vi "Inst Calibration.vi"() -> ()   [LabVIEW 2016, in "User Interface.lvlib"]
uses:
  User Interface.lvlib
  VI Name.ctl
  Calibration/Calibration.lvlib
  Calibration/Calibration Command.ctl
  Inst Calibration Data Highway.ctl
panel:
  in  "Calibration Check?":bool
  out "Status":string
  in  "Data":string[][](table)
  in  "Save":bool
  in  "Restore":bool
  out "Status":string
  in  "Exit":bool
  in  "Stop":bool
  out "error out":errorcluster
  in  "error in (no error)":errorcluster
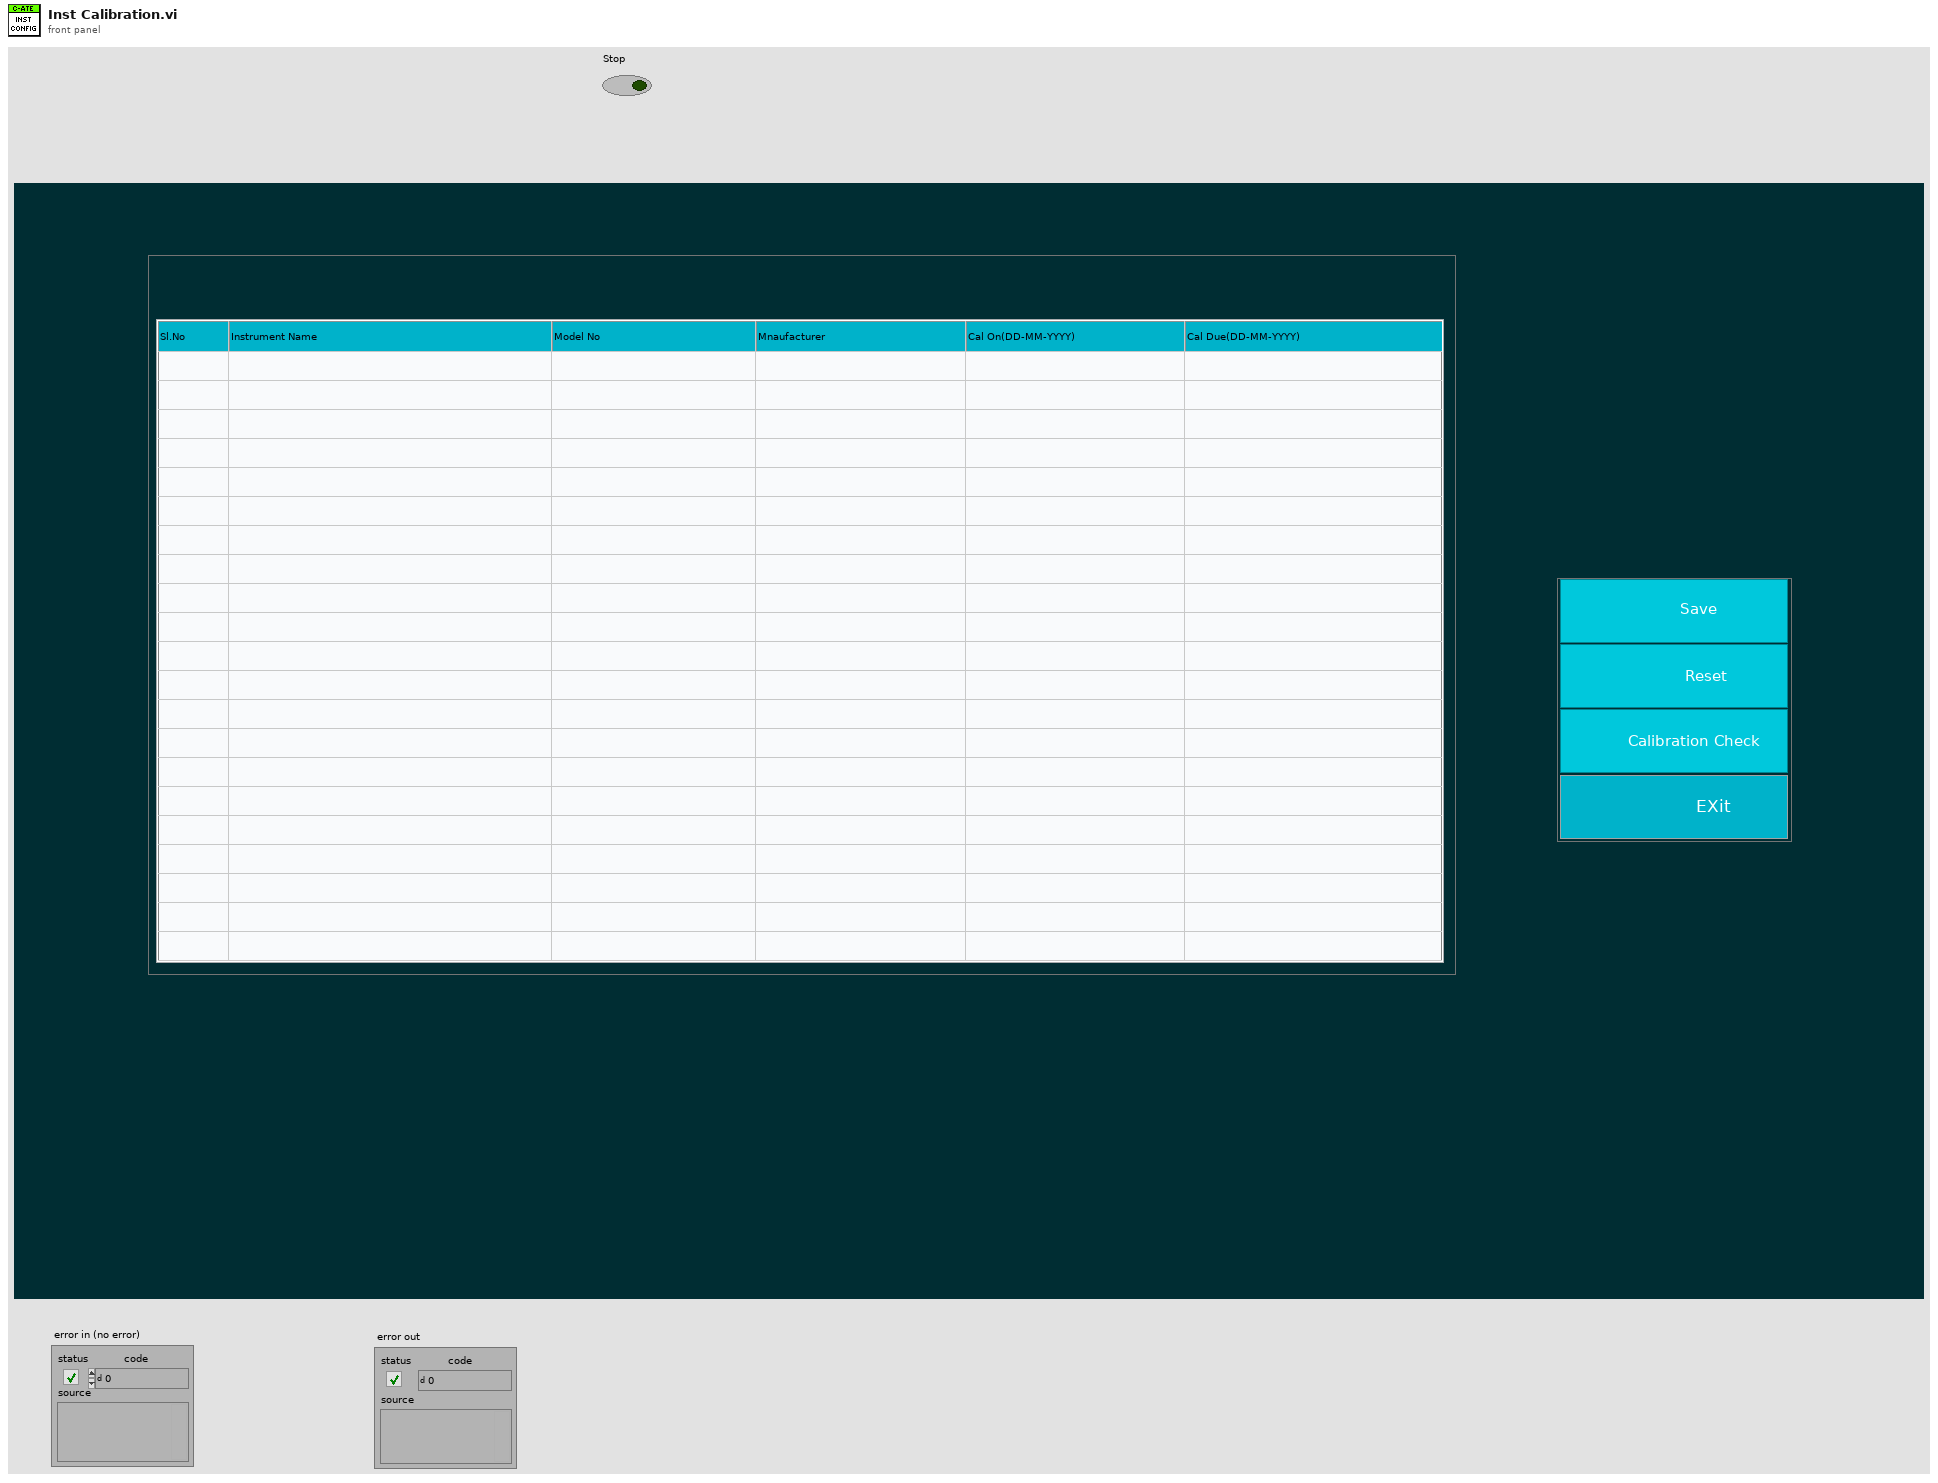
[diagram p1: front panel]
types:
  T1 = typedef "User Interface.lvlib/Inst Calibration Data Highway.ctl" = cluster{"Data":refnum<vi>, "Status":refnum<vi>, "Status":string, "Calibration Due Status":string[]}
  T2 = typedef "Calibration.lvlib/Calibration Command.ctl" = enum16{"Init", "Read", "Write", "Check Calibration", "Close"}
  T3 = typedef "User Interface.lvlib/VI Name.ctl" = enum16{"Dashboard", "Maintenance", "Recipe", "Inst Calibration", "Testing", "Report"}
  T4 = typedef "LVPoint32TypeDef.ctl" = cluster{"Horizontal":i32, "Vertical":i32}
  T5 = typedef "LVRowAndColumnTypeDef.ctl" = cluster{"Row":i32, "Column":i32}
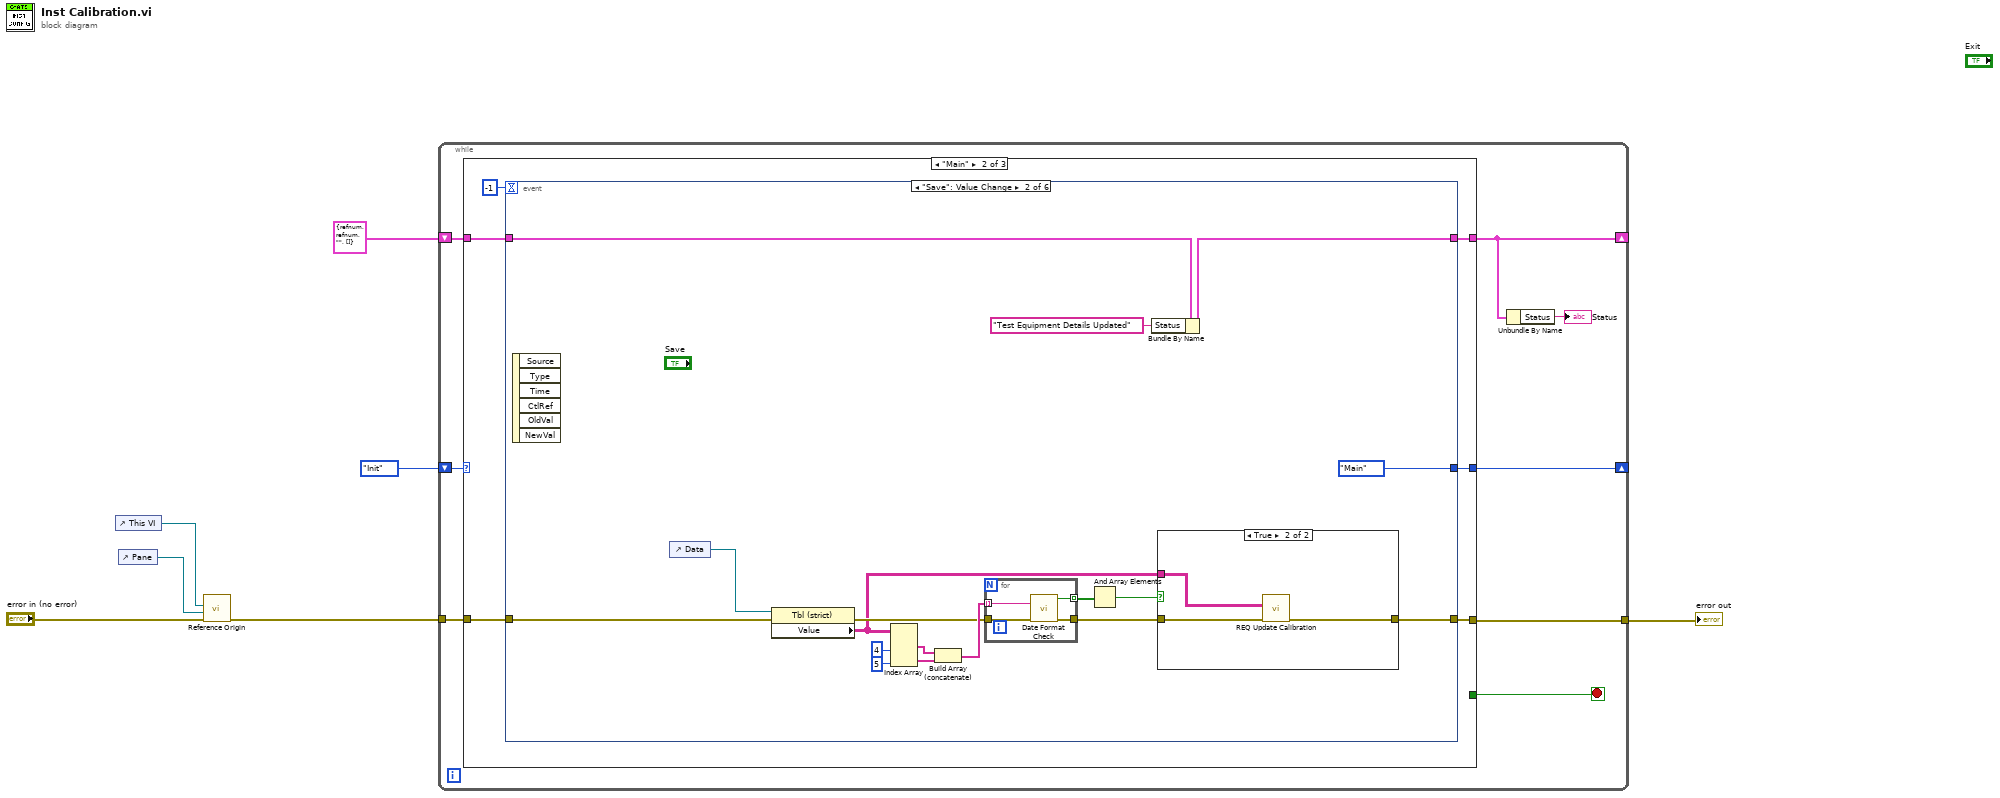
[diagram p0: block diagram]
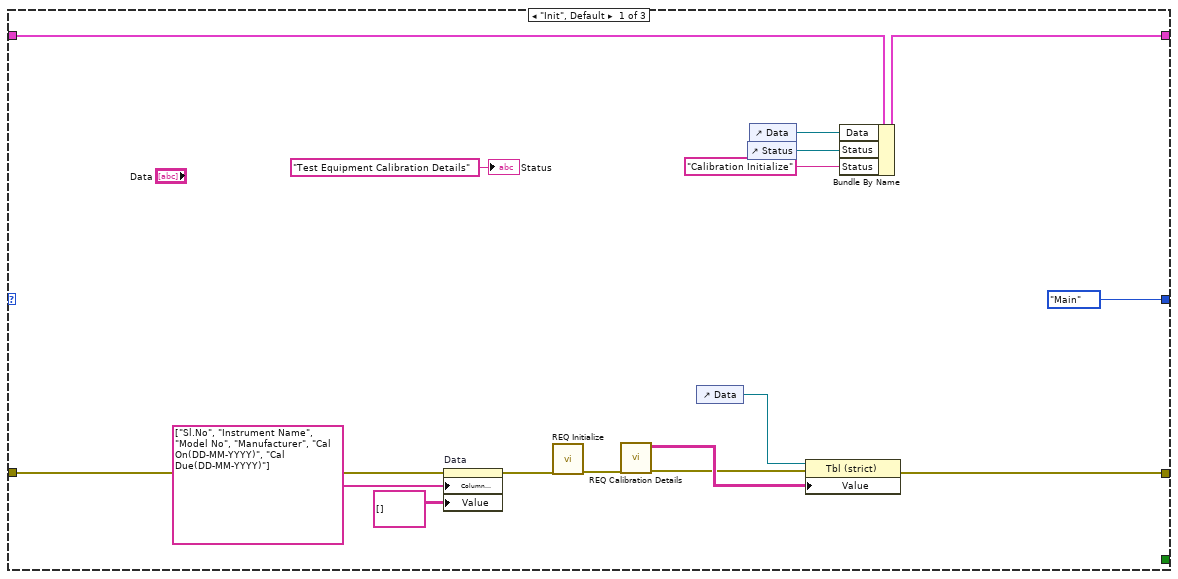
[diagram p2: hidden frame]
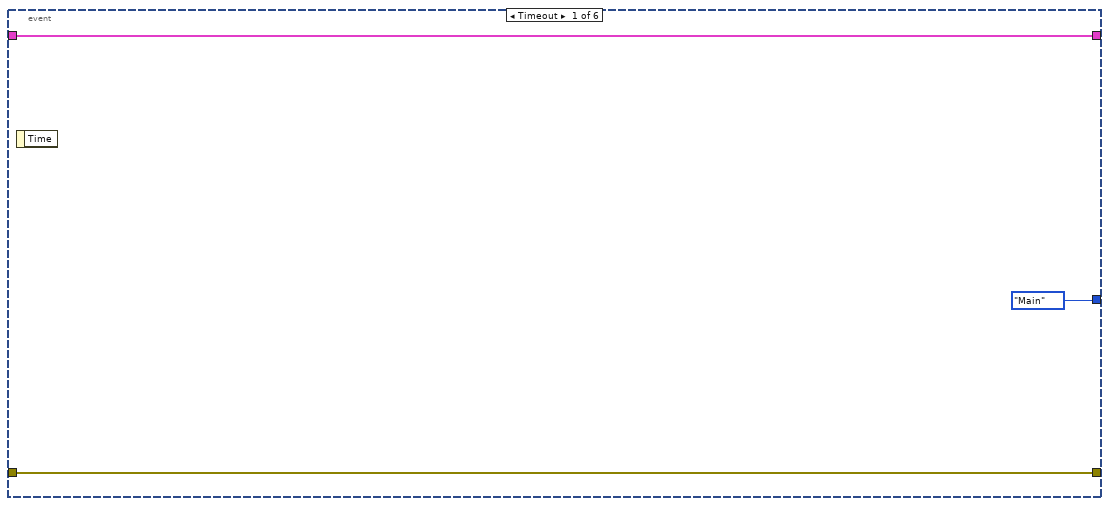
[diagram p3: hidden frame]
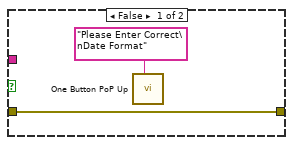
[diagram p4: hidden frame]
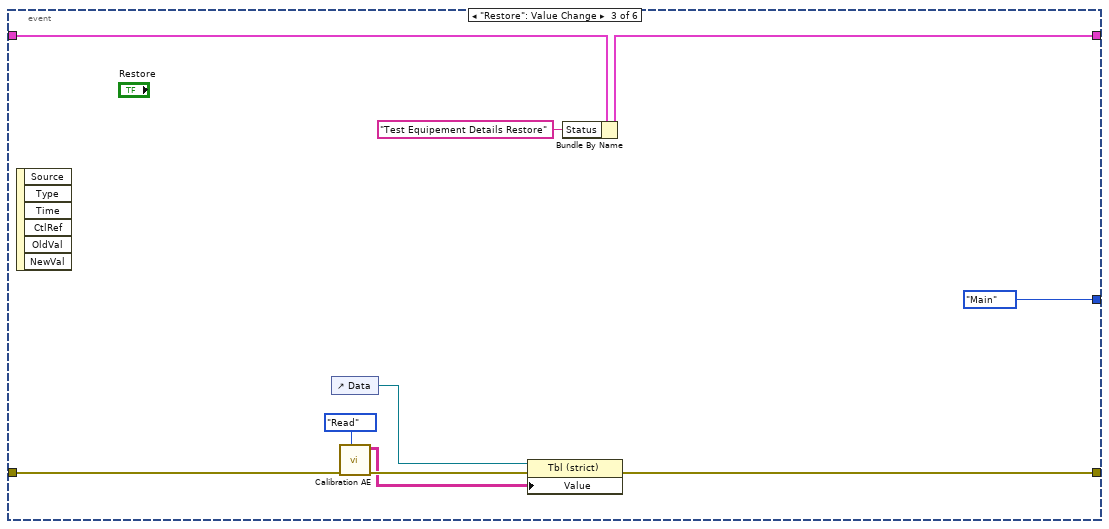
[diagram p5: hidden frame]
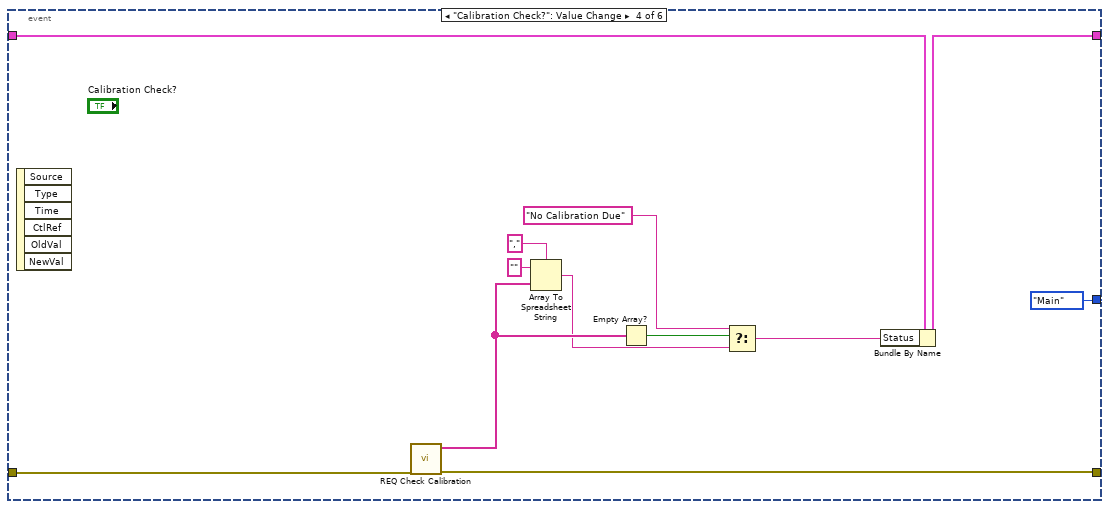
[diagram p6: hidden frame]
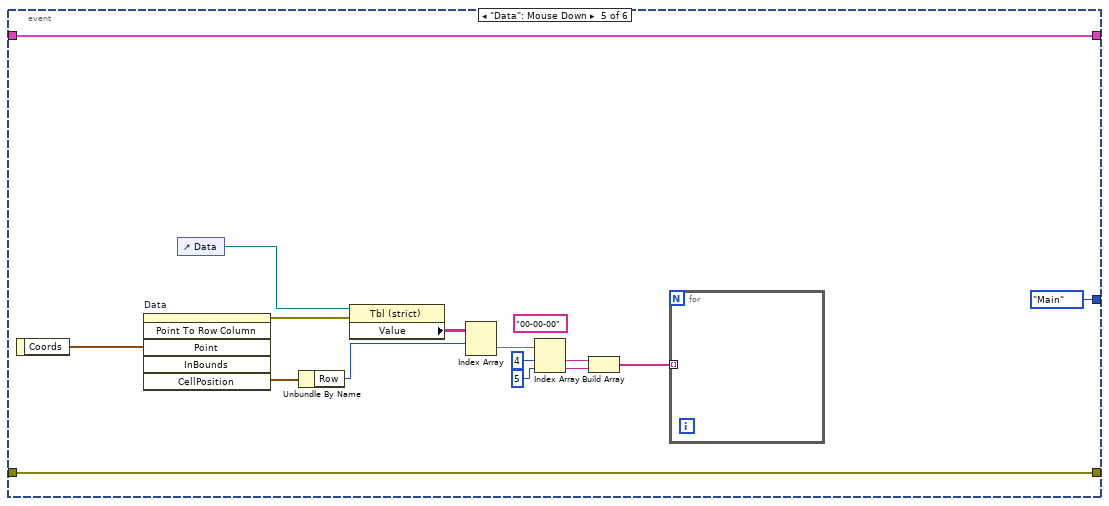
[diagram p7: hidden frame]
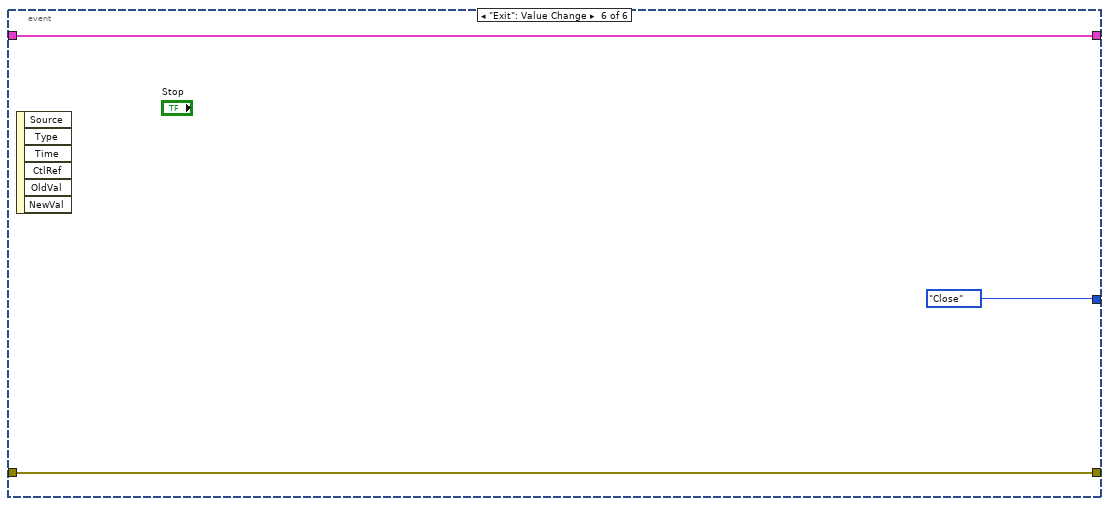
[diagram p8: hidden frame]
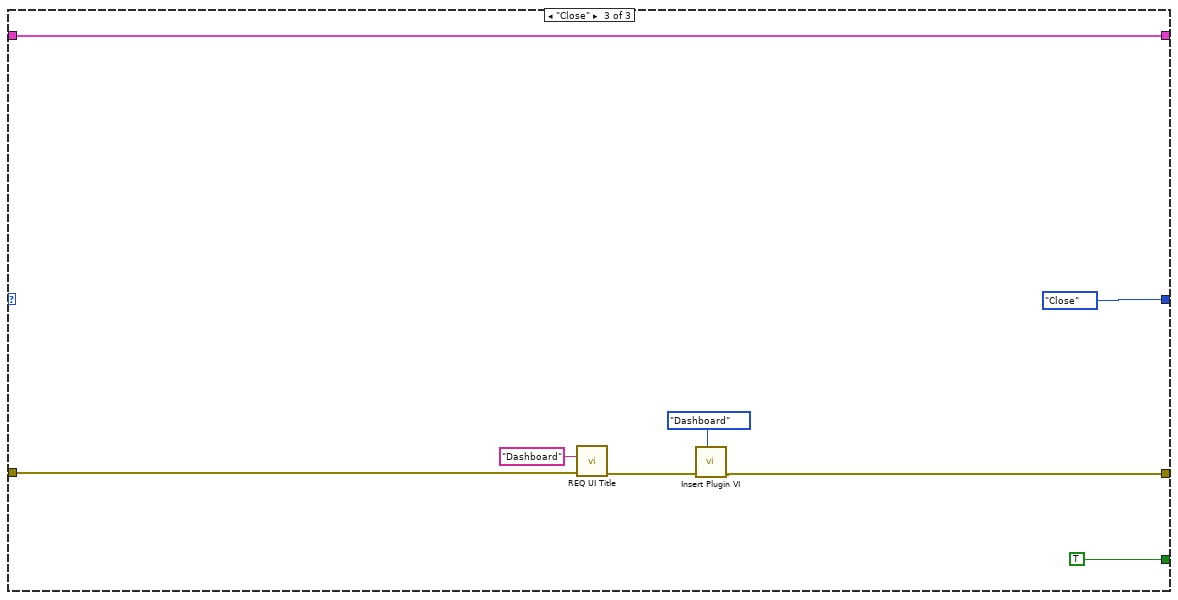
[diagram p9: hidden frame]
diagram:
  n1 = control-ref of="This VI"() -> (w6:refnum<vi>)
  n2 = control-ref of="Pane"() -> (w5:refnum<vi>)
  n3 = call "Reference Origin.vi"("error in (no error)"="error in (no error)", "Pane"=w5, "This VI"=w6) -> ("error out"=w4:errorcluster)  [unwired: 8 in]
  n4 = while {
    tunnel: w4 -> [w15]
    shift-right: [w12] -> _
    shift-left: enum16{"Init", "Main", "Close"}."Init" -> [w14]
    shift-right: [w10] -> _
    shift-left: T1 {"Data"=refnum, "Status"=refnum, "Status"="", "Calibration Due Status"=[]} -> [w13]
    tunnel: [w8] -> w1
    stop <- w11 stop-if-true
    n5 = case shown="\"Main\"" w14 {
      tunnel: w15 -> [w28 w33 w107]
      tunnel: w13 -> [w31 w36 w114]
      tunnel: [enum16{"Init", "Main", "Close"}."Main" w37 enum16{"Init", "Main", "Close"}."Close"] -> w12
      tunnel: [w30 w35 w114] -> w10
      tunnel: [_ _ TRUE] -> w11
      tunnel: [w21 w32 w108] -> w8
      frame "Init", Default {
        n6 = property on="Data" class="Tbl (strict)"(error in=w28, "Column Headers[]"=string[] ["Sl.No", "Instrument Name", "Model No", "Manufacturer", "Cal On(DD-MM-YYYY)", "Cal Due(DD-MM-YYYY)"] ("Column Header Strings[]"), "Value"=string[][] []) -> (error out=w19:errorcluster)  [unwired: 1 in, 1 out]
        n7 = call "REQ Initialize.vi"("error in"=w19) -> ("error out"=w18:errorcluster)  [unwired: 10 in]
        n8 = call "REQ Calibration Details.vi"("error in"=w18) -> ("error out"=w16:errorcluster, "Calibration Details"=w17:string[][])  [unwired: 8 in, 1 out]
        n9 = control-ref of="Data"() -> (w22:refnum<vi>)
        n10 = control-ref of="Status"() -> (w25:refnum<vi>)
        n11 = control-ref of="Data"() -> (w26:refnum<vi>)
        n12 = property class="Tbl (strict)"(reference=w22, error in=w16, "Value"=w17) -> (error out=w21:errorcluster)  [unwired: 1 out]
        n13 = Bundle By Name(cluster=w31, "Data"=w26, "Status"=w25, "Status"="Calibration Initialize") -> (w30:T1)
        "Status" <- "Test Equipment Calibration Details" ("Status")
      }
      frame "Main" {
        n14 = event shown="[1] \"Save\": Value Change" {
          selector: _ -> [_ _ _ _ _ _]
          dyn-events: _ -> [_ _ _ _ _ _]
          timeout: -1 -> [_ _ _ _ _ _]
          tunnel: [enum16{"Init", "Main", "Close"}."Main" enum16{"Init", "Main", "Close"}."Main" enum16{"Init", "Main", "Close"}."Main" enum16{"Init", "Main", "Close"}."Main" enum16{"Init", "Main", "Close"}."Main" enum16{"Init", "Main", "Close"}."Close"] -> w37
          tunnel: w36 -> [w40 w57 w76 w88 w101 w106]
          tunnel: [w40 w53 w69 w78 w101 w106] -> w35
          tunnel: w33 -> [w38 w54 w73 w86 w92 w104]
          tunnel: [w38 w51 w70 w85 w92 w104] -> w32
          event Timeout {
            n15 = event-data() -> ()  [unwired: 1 in, 1 out]
          }
          event "Save": Value Change {
            n16 = event-data() -> ()  [unwired: 1 in, 6 out]
            n17 = control-ref of="Data"() -> (w55:refnum<vi>)
            n18 = property class="Tbl (strict)"(reference=w55, error in=w54) -> (error out=w45:errorcluster, "Value"=w41:string[][])  [unwired: 1 out]
            n19 = Index Array(array=w41, index (col) #1=4 ("disabled index (col)"), index (col) #2=5 ("index (col)")) -> (element #1=w48:string[], element #2=w47:string[])  [unwired: 2 in]
            n20 = Build Array (concatenate)(w48, w47) -> (w46:string[])
            n21 = for {
              tunnel: w46 -> [w66] mode=indexing
              tunnel: w45 -> [w65]
              tunnel: [w64] -> w42
              tunnel: [w63] -> w44 mode=indexing
              n22 = call "Date Format Check.vi"("error in (no error)"=w65, "Formated Date"=w66) -> ("error out"=w64:errorcluster, "Formated?"=w63:bool)  [unwired: 8 in]
            }
            n23 = And Array Elements(Boolean array=w44) -> (logical AND=w43:bool)
            n24 = Bundle By Name(cluster=w57, "Status"="Test Equipment Details Updated") -> (w53:T1)
            n25 = case shown="True" w43 {
              tunnel: [w58 w62] -> w51
              tunnel: w42 -> [w58 w60]
              tunnel: w41 -> [_ w61]
              frame False {
                n26 = call "One Button PoP Up.vi"("Message In"="Please Enter Correct\nDate Format") -> ()  [unwired: 11 in]
              }
              frame True {
                n27 = call "REQ Update Calibration.vi"("error in"=w60, "Calibration Details In"=w61) -> ("error out"=w62:errorcluster)  [unwired: 9 in]
              }
            }
          }
          event "Restore": Value Change {
            n28 = event-data() -> ()  [unwired: 1 in, 6 out]
            n29 = control-ref of="Data"() -> (w74:refnum<vi>)
            n30 = call "Calibration AE.vi"("Command"=Calibration_Command."Read", "error in (no error)"=w73) -> ("error out"=w72:errorcluster, "Inst Details Out"=w71:string[][])  [unwired: 7 in, 1 out]
            n31 = property class="Tbl (strict)"(reference=w74, error in=w72, "Value"=w71) -> (error out=w70:errorcluster)  [unwired: 1 out]
            n32 = Bundle By Name(cluster=w76, "Status"="Test Equipement Details Restore") -> (w69:T1)
          }
          event "Calibration Check?": Value Change {
            n33 = event-data() -> ()  [unwired: 1 in, 6 out]
            n34 = call "REQ Check Calibration.vi"("error in"=w86) -> ("error out"=w85:errorcluster, "Calibration Due Msg"=w82:string[])  [unwired: 8 in, 1 out]
            n35 = Array To Spreadsheet String(delimiter (Tab)=",", array=w82, 3:"" ("format string")) -> (spreadsheet string=w80:string)
            n36 = Empty Array?(array=w82) -> (empty?=w81:bool)
            n37 = Select(t="No Calibration Due", s=w81, f=w80) -> (s? t:f=w77:string)
            n38 = Bundle By Name(cluster=w88, "Status"=w77) -> (w78:T1)
          }
          event "Data": Mouse Down {
            (unwired) "00-00-00"
            n39 = event-data() -> ("Coords"=w103:T4)  [unwired: 1 in]
            n40 = invoke on="Data" class="Tbl (strict)" method="Point To Row Column"("Point"=w103) -> (error out=w99:errorcluster, "CellPosition"=w102:T5)  [unwired: 5 in, 4 out]
            n41 = control-ref of="Data"() -> (w100:refnum<vi>)
            n42 = Unbundle By Name(w102) -> ("Row"=w97:i32)
            n43 = property class="Tbl (strict)"(reference=w100, error in=w99) -> ("Value"=w98:string[][])  [unwired: 2 out]
            n44 = Index Array(array=w98, index (row)=w97) -> (element=w96:string[])  [unwired: 1 in]
            n45 = Index Array(array=w96, index #1=4 ("index"), index #2=5 ("index")) -> (element #1=w91:string, element #2=w90:string)
            n46 = Build Array(w91, w90) -> (w89:string[])
            n47 = for {
              tunnel: w89 -> [_] mode=indexing
            }
          }
          event "Exit": Value Change {
            n48 = event-data() -> ()  [unwired: 1 in, 6 out]
          }
        }
      }
      frame "Close" {
        n49 = call "REQ UI Title.vi"("error in"=w107, "UI Title"="Dashboard" ("ATE Title")) -> ("error out"=w109:errorcluster)  [unwired: 9 in]
        n50 = call "Insert Plugin VI.vi"("VI Name"=VI_Name."Dashboard", "error in (no error)"=w109) -> ("error out"=w108:errorcluster)  [unwired: 9 in]
      }
    }
    n51 = Unbundle By Name(w10) -> ("Status"=→"Status":string)
  }
  "error out" <- w1
